vi "EventStructureLiftDev.vi"() -> ()   [LabVIEW 2016]
uses:
  <vilib>/myRIO/Instrument Drivers/Onboard IO/DIO/typedefs/DIO Reference.ctl
  <vilib>/myRIO/Common/Instrument Driver Framework/Utilities/typedefs/myRIO Generic Hardware Reference.ctl
  <vilib>/myRIO/Common/Instrument Driver Framework/Utilities/typedefs/Hardware Version Enum.ctl
  <vilib>/myRIO/Common/Instrument Driver Framework/Utilities/typedefs/myRIO v1.0 Reference.ctl
  <vilib>/myRIO/Common/Instrument Driver Framework/Utilities/typedefs/Generic FPGA Reference.ctl
  <vilib>/myRIO/Common/Instrument Driver Framework/myRIO v1.0/DIO/typedefs/DIO Channels List.ctl
  <vilib>/myRIO/Common/Instrument Driver Framework/myRIO v1.0/DIO/typedefs/DIO Channels Enum.ctl
  <vilib>/userdefined/High Color/nirio_resource_hc.ctl
  <vilib>/myRIO/Common/Instrument Driver Framework/Utilities/vis/Is FPGA Ref Available.vi
  <vilib>/myRIO/Common/Instrument Driver Framework/roboRIO v1.0/DIO/vis/roboRIO v1.0 Open DIO.vi
  <vilib>/myRIO/Instrument Drivers/Onboard IO/DIO/vis/Write.vi
  <vilib>/myRIO/Instrument Drivers/Onboard IO/DIO/vis/Read.vi
  <vilib>/myRIO/Common/Instrument Driver Framework/Utilities/vis/Validate Channels.vi
  <vilib>/myRIO/Common/Instrument Driver Framework/roboRIO v1.0/DIO/vis/roboRIO v1.0 Reserve DIO.vi
  <vilib>/myRIO/Common/Instrument Driver Framework/roboRIO v1.0/DIO/vis/roboRIO v1.0 Build MUX Configuration DIO.vi
  <vilib>/myRIO/Common/Instrument Driver Framework/roboRIO v1.0/Resource Manager/vis/roboRIO v1.0 Reserve Channel List.vi
  <vilib>/myRIO/Common/Instrument Driver Framework/roboRIO v1.0/Resource Manager/vis/roboRIO v1.0 Create Configuration List.vi
  <vilib>/myRIO/Common/Instrument Driver Framework/roboRIO v1.0/Resource Manager/vis/roboRIO v1.0 Reserve Channel.vi
  <vilib>/myRIO/Common/Instrument Driver Framework/roboRIO v1.0/Resource Manager/vis/roboRIO v1.0 Unreserve Channel.vi
  <vilib>/myRIO/Common/Instrument Driver Framework/roboRIO v1.0/Resource Manager/vis/roboRIO v1.0 Build Mutex Name.vi
  UnicornMain/GlobalVI.vi
  <vilib>/Utility/VariantDataType/GetNumericInfo.vi
  builds/UnicornMain/UnicornRIO1/ROS for LabVIEW/home/lvuser/natinst/bin/vi.lib/Utility/error.llb/Error Cluster From Error Code.vi
  <vilib>/myRIO/Common/Instrument Driver Framework/roboRIO v1.0/roboRIO v1.0 Open.vi
  <vilib>/myRIO/Common/Instrument Driver Framework/Utilities/vis/IO Manager.vi
  <vilib>/myRIO/Common/Instrument Driver Framework/Utilities/vis/Configuration Manager.vi
  <vilib>/myRIO/Common/Instrument Driver Framework/roboRIO v1.0/Resource Manager/vis/roboRIO v1.0 Configure IO.vi
  <vilib>/myRIO/Common/Instrument Driver Framework/myRIO v1.0/myRIO v1.0 Close.vi
  <vilib>/myRIO/Common/Instrument Driver Framework/roboRIO v1.0/DIO/vis/roboRIO v1.0 Write DIO.vi
  <vilib>/myRIO/Common/Instrument Driver Framework/roboRIO v1.0/DIO/vis/roboRIO v1.0 Read DIO.vi
  <vilib>/myRIO/Express VI/Onboard IO/DO/DO Express VI.xnode
  <vilib>/myRIO/Instrument Drivers/Onboard IO/DIO/vis/myRIO DIO Open.xnode
  <vilib>/myRIO/Express VI/Onboard Devices/LED/LED Express VI.xnode
  <vilib>/myRIO/Express VI/Onboard IO/DI/DI Express VI.xnode
  <vilib>/myRIO/Instrument Drivers/Onboard IO/DIO/DIO.lvlib
panel:
  out "UnloadBin":bool
  out "CancelBin":bool
  out "B/DIO7 (Pin 25) 2":bool
  out "B/DIO10 (Pin 31) 2":bool
  out "B/DIO10 (Pin 31) - Sensor 5\nBackwards 3":bool
  out "B/DIO7 (Pin 25) - Sensor 2 - Down 2":bool
  out "B/DIO9 (Pin 29) - Sensor4 - Forward 2":bool
  out "B/DIO8 (Pin 27) - Sensor3 - Up 2":bool
  out "LoadBin":bool
  out "B/DIO7 (Pin 25) - Sensor2 - Down 2":bool
  out "B/DIO10 (Pin 31) - Sensor 5\nBackwards 2":bool
  out "B/DIO8 (Pin 27) - Sensor 3 - Up 2":bool
  out "B/DIO9 (Pin 29) - Sensor 4 - Forward 2":bool
  out "StopBin":bool
  out "timeoutCounter":u32
  out "timeoutError":bool
  out "timerCount":u32
  out "liftState":i32
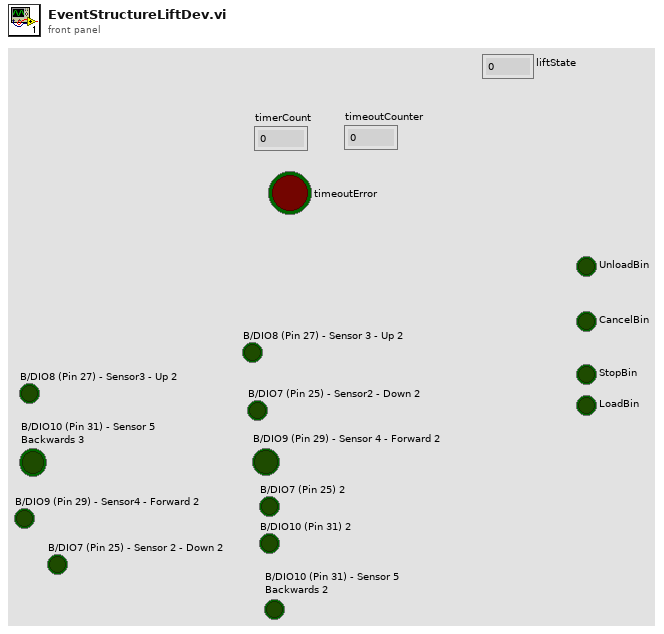
[diagram p1: front panel]
types:
  T1 = typedef "DIO.lvlib/DIO Reference.ctl" = cluster{"myRIO Reference":T2, "DIO Channels List":T6}
  T2 = typedef "myRIO Generic Hardware Reference.ctl" = cluster{"myRIO Model":T3, "myRIO Hardware Reference":T4}
  T3 = typedef "Hardware Version Enum.ctl" = enum16{"Unknown", "myRIO-1900", "myRIO-1950", "roboRIO", "NI ELVIS RIO CM"}
  T4 = typedef "myRIO v1.0 Reference.ctl" = cluster{"Generic FPGA Reference":T5, "Allow multiple opens":bool}
  T5 = typedef "Generic FPGA Reference.ctl" = refnum<k20>
  T6 = typedef "DIO Channels List.ctl" = T7[]
  T7 = typedef "DIO Channels Enum.ctl" = enum16{"Not Connected", "C/DIO0", "C/DIO1", "C/DIO2", "C/DIO3", "C/DIO4", "C/DIO5", "C/DIO6", "C/DIO7", "A/DIO0", "A/DIO1", "A/DIO2", "A/DIO3", "A/DIO4", "A/DIO5", "A/DIO6", "A/DIO7", "A/DIO8", "A/DIO9", "A/DIO10", "A/DIO11", "A/DIO12", "A/DIO13", "A/DIO14", "A/DIO15", "B/DIO0", "B/DIO1", "B/DIO2", "B/DIO3", "B/DIO4", "B/DIO5", "B/DIO6", "B/DIO7", "B/DIO8", "B/DIO9", "B/DIO10", "B/DIO11", "B/DIO12", "B/DIO13", "B/DIO14", "B/DIO15", "LED0", "LED1", "LED2", "LED3", "Button0", "DIO/DIO0", "DIO/DIO1", "DIO/DIO2", "DIO/DIO3", "DIO/DIO4", "DIO/DIO5", "DIO/DIO6", "DIO/DIO7", "DIO/DIO8", "DIO/DIO9", "SPI/CS0", "SPI/CS1", "SPI/CS2", "SPI/CS3", "LED RADIO (Green)", "LED RADIO (Red)", "LED COMM (Green)", "LED COMM (Red)", "LED MODE (Green)", "LED MODE (Red)"}
  T8 = typedef "nirio_resource_hc.ctl" = tag
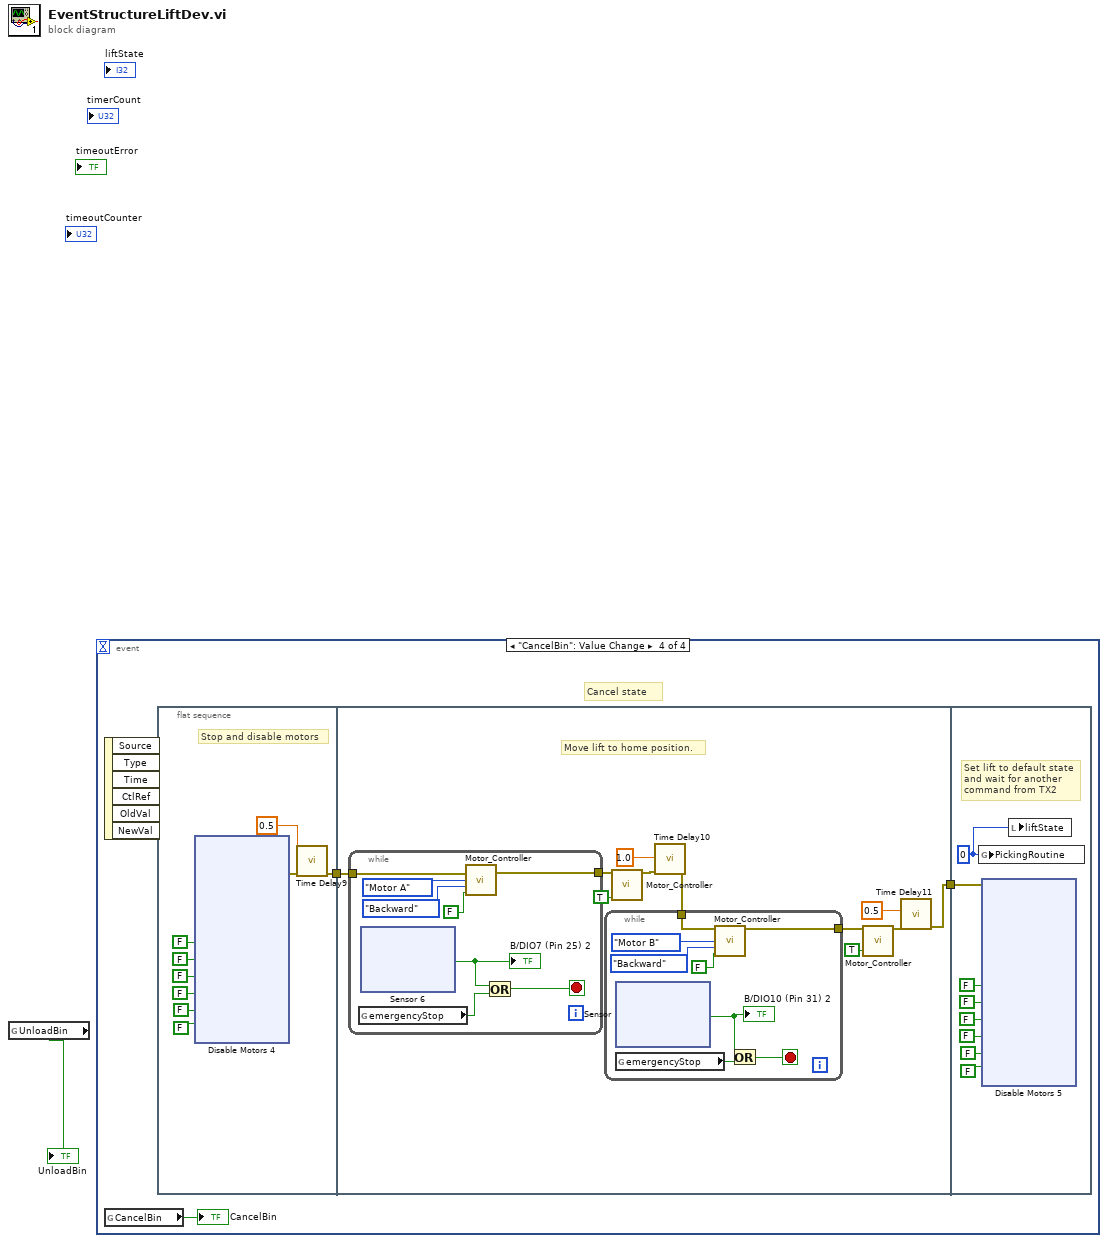
[diagram p0: block diagram]
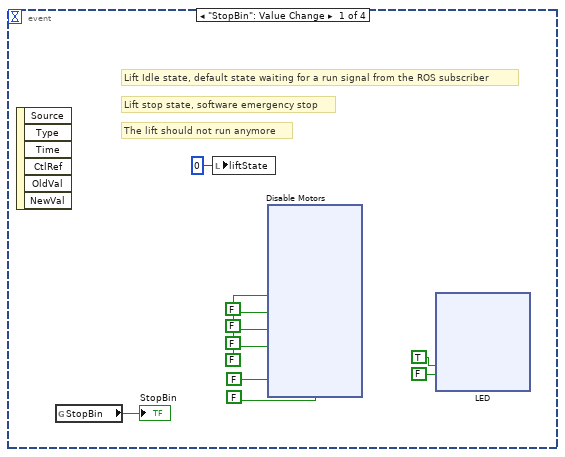
[diagram p2: hidden frame]
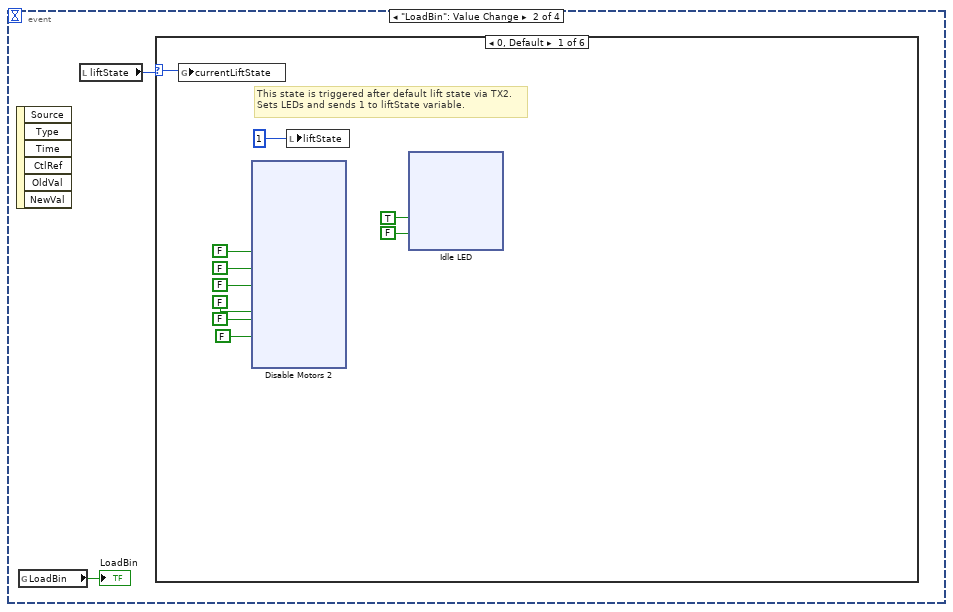
[diagram p3: hidden frame]
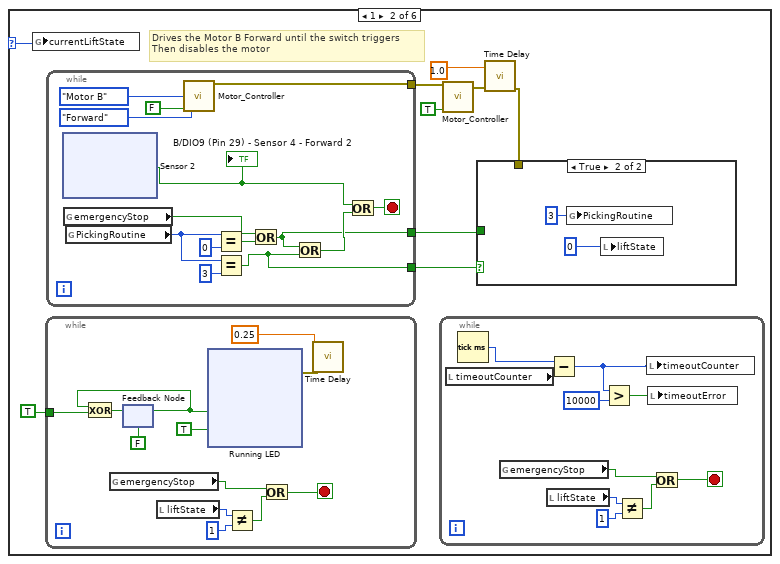
[diagram p4: hidden frame]
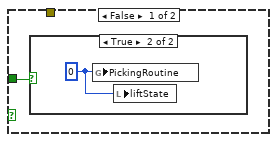
[diagram p5: hidden frame]
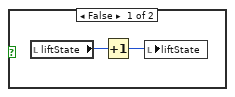
[diagram p6: hidden frame]
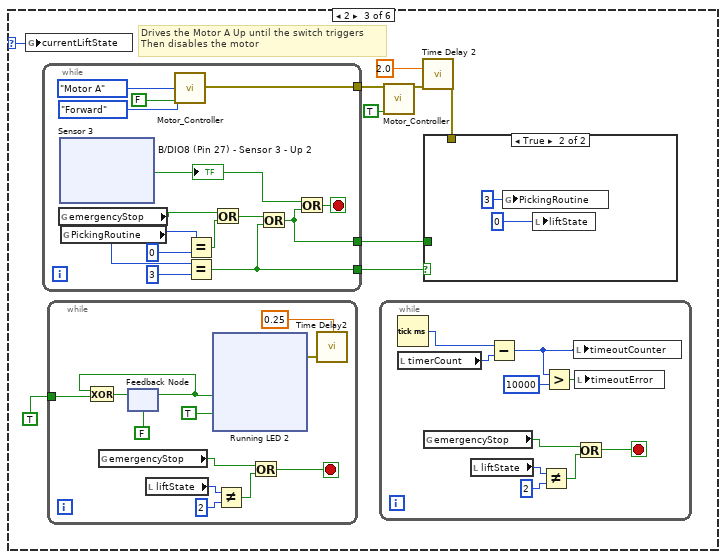
[diagram p7: hidden frame]
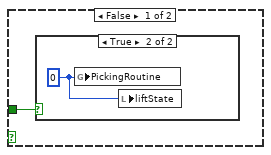
[diagram p8: hidden frame]
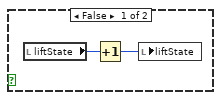
[diagram p9: hidden frame]
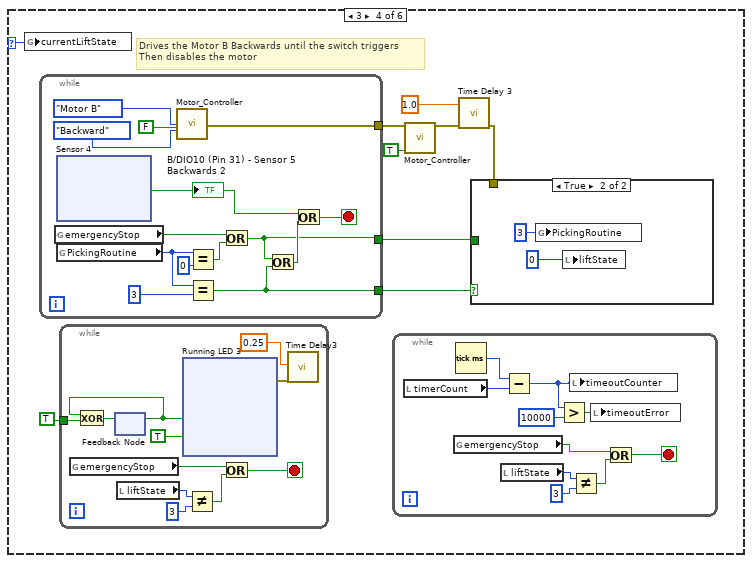
[diagram p10: hidden frame]
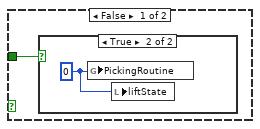
[diagram p11: hidden frame]
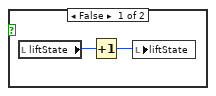
[diagram p12: hidden frame]
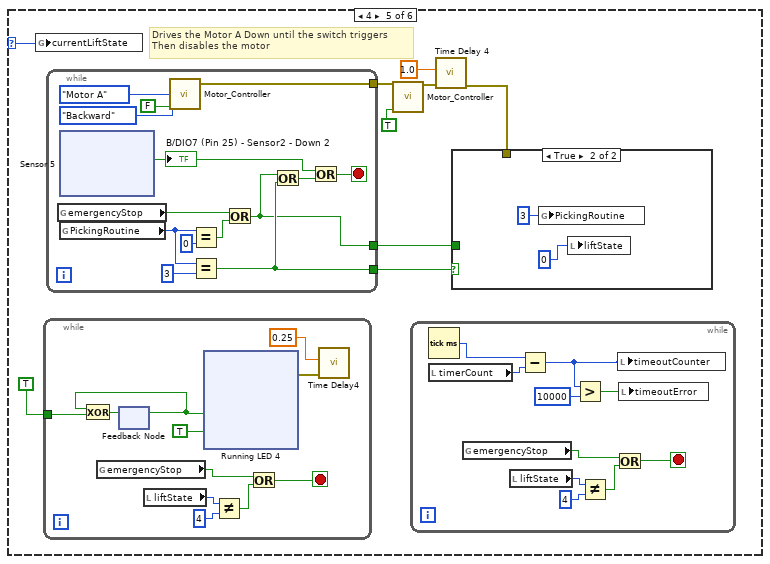
[diagram p13: hidden frame]
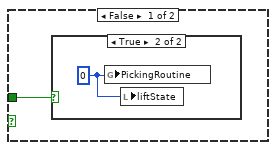
[diagram p14: hidden frame]
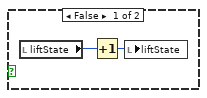
[diagram p15: hidden frame]
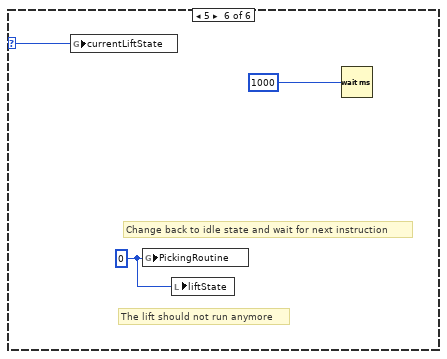
[diagram p16: hidden frame]
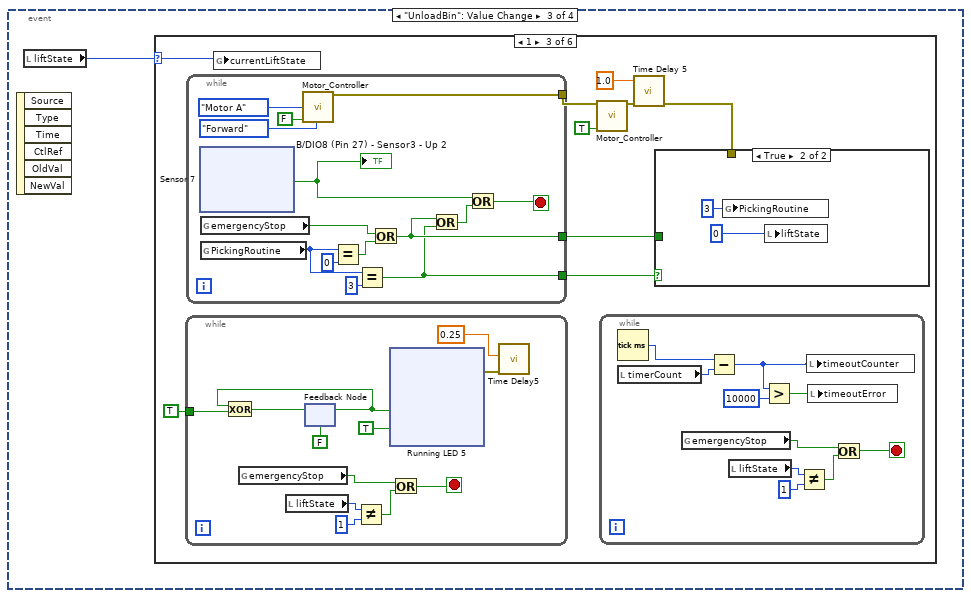
[diagram p17: hidden frame]
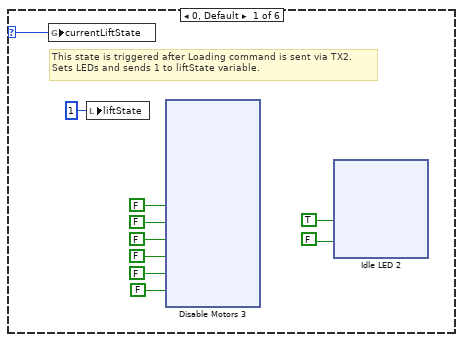
[diagram p18: hidden frame]
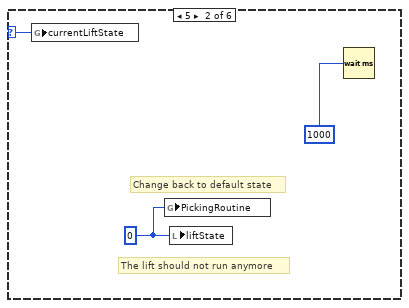
[diagram p19: hidden frame]
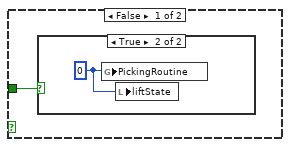
[diagram p20: hidden frame]
diagram:
  n1 = global read "GlobalVI.vi" "UnloadBin"() -> (→"UnloadBin":bool)
  n2 = event shown="[3] \"CancelBin\": Value Change" {
    selector: _ -> [_ _ _ _]
    dyn-events: _ -> [_ _ _ _]
    timeout: _ -> [_ _ _ _]
    event "StopBin": Value Change {
      # "Lift stop state, software emergency stop"
      # "Lift Idle state, default state waiting for a run signal from the ROS subscriber"
      # "The lift should not run anymore"
      n3 = event-data() -> ()  [unwired: 1 in, 6 out]
      n4 = global read "GlobalVI.vi" "StopBin"() -> (→"StopBin":bool)
      n5 = local write "liftState"(0 ("liftState")) -> ()
      n6 = xnode "Disable Motors"("IN1 (B/DIO1 (Pin 13))"=FALSE ("IN1 (B/DIO0 (Pin 11))"), "IN2 (B/DIO2 (Pin 15))"=FALSE ("IN2 (B/DIO1 (Pin 13))"), "IN3 (B/DIO4 (Pin 19))"=FALSE ("IN3 (B/DIO2 (Pin 15))"), "IN4 (B/DIO3 (Pin 17))"=FALSE, "ENABLE A (B/DIO0 (Pin 11))"=FALSE ("ENABLE A (B/DIO13 (Pin 26))"), "ENABLE B (B/DIO5 (Pin 21))"=FALSE ("ENABLE B (B/DIO8 (Pin 27))")) -> ()  [unwired: 1 in, 1 out]
      n7 = xnode "LED"("COMM (Green)"=TRUE, "COMM (Red)"=FALSE) -> ()  [unwired: 1 in, 1 out]
    }
    event "LoadBin": Value Change {
      n8 = event-data() -> ()  [unwired: 1 in, 6 out]
      n9 = global read "GlobalVI.vi" "LoadBin"() -> (→"LoadBin":bool)
      n10 = local read "liftState"() -> (w88:i32)
      n11 = case shown="0, Default" w88 {
        selector: w88 -> [w96 w179 w302 w423 w544 w664]
        frame 0, Default {
          # "This state is triggered after default lift state via TX2. \nSets LEDs and sends 1 to liftState variable."
          n12 = global write "GlobalVI.vi" "currentLiftState"(w96) -> ()
          n13 = xnode "Disable Motors 2"("IN1 (B/DIO1 (Pin 13))"=FALSE ("IN1 (B/DIO0 (Pin 11))"), "IN2 (B/DIO2 (Pin 15))"=FALSE ("IN2 (B/DIO1 (Pin 13))"), "IN3 (B/DIO4 (Pin 19))"=FALSE ("IN3 (B/DIO2 (Pin 15))"), "IN4 (B/DIO3 (Pin 17))"=FALSE, "ENABLE A (B/DIO0 (Pin 11))"=FALSE ("ENABLE A (B/DIO13 (Pin 26))"), "ENABLE B (B/DIO5 (Pin 21))"=FALSE ("ENABLE B (B/DIO8 (Pin 27))")) -> ()  [unwired: 1 in, 1 out]
          n14 = local write "liftState"(1 ("liftState")) -> ()
          n15 = xnode "Idle LED"("CommG"=TRUE, "CommR"=FALSE ("CommG")) -> ()  [unwired: 1 in, 1 out]
        }
        frame 1 {
          # "Drives the Motor B Forward until the switch triggers\nThen disables the motor"
          n16 = global write "GlobalVI.vi" "currentLiftState"(w179) -> ()
          n17 = while {
            tunnel: TRUE ("COMM (Red)") -> [w212]
            stop <- w202 stop-if-true
            n18 = global read "GlobalVI.vi" "emergencyStop"() -> (w203:bool)
            n19 = feedback #1(FALSE) -> (w210:bool)
            n20 = Exclusive Or(1:w212, 2:w210) -> (0:w211:bool)
            n21 = feedback-in #1(w211) -> ()
            n22 = local read "liftState"() -> (w205:i32)
            n23 = xnode "Running LED"("CommG"=w210, "CommR"=TRUE) -> ("error out"=w207:errorcluster)  [unwired: 1 in]
            n24 = Not Equal?(x=w205, y=1 ("liftState")) -> (x != y?=w204:bool)
            n25 = Or(x=w203, y=w204) -> (x .or. y?=w202:bool)
            n26 = call "Time Delay"("error in (no error)"=w207, "Delay Time (s)"=0.25) -> ()  [unwired: 9 in, 1 out]
          }
          n27 = while {
            tunnel: [w261] -> w180
            tunnel: [w250] -> w177
            tunnel: [w249] -> w178
            stop <- w262 stop-if-true
            n28 = xnode "Sensor 2"() -> ("B/DIO9 (Pin 29)"=w257:bool)  [unwired: 1 in, 1 out]
            "B/DIO9 (Pin 29) - Sensor 4 - Forward 2" <- w257
            n29 = global read "GlobalVI.vi" "emergencyStop"() -> (w255:bool)
            n30 = global read "GlobalVI.vi" "PickingRoutine"() -> (w252:i32)
            n31 = call "Motor_Controller.vi"("motorSelect"=enum16{"Motor A", "Motor B"}."Motor B", "direction"=enum16{"Forward", "Backward"}."Forward", "stopMotors"=FALSE) -> ("error out"=w261:errorcluster)  [unwired: 12 in]
            n32 = Equal?(x=w252, y=0) -> (x = y?=w254:bool)
            n33 = Equal?(x=w252, y=3) -> (x = y?=w249:bool)
            n34 = Or(x=w255, y=w254) -> (x .or. y?=w250:bool)
            n35 = Or(x=w250, y=w249) -> (x .or. y?=w251:bool)
            n36 = Or(x=w257, y=w251) -> (x .or. y?=w262:bool)
          }
          n37 = while {
            stop <- w194 stop-if-true
            n38 = local read "timeoutCounter"() -> (w199:u32)
            n39 = Tick Count (ms)() -> (millisecond timer value=w200:u32)
            n40 = global read "GlobalVI.vi" "emergencyStop"() -> (w198:bool)
            n41 = local read "liftState"() -> (w196:i32)
            n42 = Subtract(x=w200, y=w199) -> (x-y=w191:u32)
            n43 = Greater?(x=w191, y=u32 10000) -> (0:w192:bool)
            n44 = Not Equal?(x=w196, y=1 ("liftState")) -> (x != y?=w197:bool)
            n45 = local write "timeoutCounter"(w191) -> ()
            n46 = local write "timeoutError"(w192) -> ()
            n47 = Or(x=w198, y=w197) -> (x .or. y?=w194:bool)
          }
          n48 = call "Motor_Controller.vi"("error in (no error)"=w180, "stopMotors"=TRUE) -> ("error out"=w181:errorcluster)  [unwired: 13 in]
          n49 = call "Time Delay"("error in (no error)"=w181, "Delay Time (s)"=1.0) -> ("error out"=w176:errorcluster)  [unwired: 9 in]
          n50 = case shown="True" w178 {
            tunnel: w177 -> [w185 _]
            tunnel: w176 -> [_ _]
            frame False {
              n51 = case shown="True" w185 {
                frame False {
                  n52 = local read "liftState"() -> (w187:i32)
                  n53 = Increment(x=w187) -> (x+1=w186:i32)
                  n54 = local write "liftState"(w186) -> ()
                }
                frame True {
                  w188 = 0 ("liftState")
                  n55 = global write "GlobalVI.vi" "PickingRoutine"(w188) -> ()
                  n56 = local write "liftState"(w188) -> ()
                }
              }
            }
            frame True {
              n57 = global write "GlobalVI.vi" "PickingRoutine"(3 ("PickingRoutine")) -> ()
              n58 = local write "liftState"(0 ("liftState")) -> ()
            }
          }
        }
        frame 2 {
          # "Drives the Motor A Up until the switch triggers\nThen disables the motor"
          n59 = global write "GlobalVI.vi" "currentLiftState"(w302) -> ()
          n60 = while {
            tunnel: [w382] -> w301
            tunnel: [w372] -> w300
            tunnel: [w371] -> w299
            stop <- w379 stop-if-true
            n61 = global read "GlobalVI.vi" "emergencyStop"() -> (w378:bool)
            n62 = xnode "Sensor 3"() -> ("Upwards (B/DIO8 (Pin 27))"=w380:bool)  [unwired: 1 in, 1 out]
            "B/DIO8 (Pin 27) - Sensor 3 - Up 2" <- w380
            n63 = global read "GlobalVI.vi" "PickingRoutine"() -> (w374:i32)
            n64 = call "Motor_Controller.vi"("motorSelect"=enum16{"Motor A", "Motor B"}."Motor A", "direction"=enum16{"Forward", "Backward"}."Forward", "stopMotors"=FALSE) -> ("error out"=w382:errorcluster)  [unwired: 12 in]
            n65 = Equal?(x=w374, y=0) -> (x = y?=w377:bool)
            n66 = Equal?(x=w374, y=3) -> (x = y?=w372:bool)
            n67 = Or(x=w378, y=w377) -> (x .or. y?=w373:bool)
            n68 = Or(x=w373, y=w372) -> (x .or. y?=w371:bool)
            n69 = Or(x=w380, y=w371) -> (x .or. y?=w379:bool)
          }
          n70 = while {
            tunnel: TRUE ("COMM (Red)") -> [w334]
            stop <- w324 stop-if-true
            n71 = global read "GlobalVI.vi" "emergencyStop"() -> (w325:bool)
            n72 = feedback #2(FALSE) -> (w332:bool)
            n73 = Exclusive Or(1:w334, 2:w332) -> (0:w333:bool)
            n74 = feedback-in #2(w333) -> ()
            n75 = local read "liftState"() -> (w327:i32)
            n76 = xnode "Running LED 2"("CommG"=w332, "CommR"=TRUE) -> ("error out"=w329:errorcluster)  [unwired: 1 in]
            n77 = Not Equal?(x=w327, y=2 ("liftState")) -> (x != y?=w326:bool)
            n78 = Or(x=w325, y=w326) -> (x .or. y?=w324:bool)
            n79 = call "Time Delay2"("error in (no error)"=w329, "Delay Time (s)"=0.25) -> ()  [unwired: 9 in, 1 out]
          }
          n80 = while {
            stop <- w316 stop-if-true
            n81 = Tick Count (ms)() -> (millisecond timer value=w322:u32)
            n82 = local read "timerCount"() -> (w321:u32)
            n83 = global read "GlobalVI.vi" "emergencyStop"() -> (w320:bool)
            n84 = local read "liftState"() -> (w318:i32)
            n85 = Subtract(x=w322, y=w321) -> (x-y=w313:u32)
            n86 = Not Equal?(x=w318, y=2 ("liftState")) -> (x != y?=w319:bool)
            n87 = Greater?(x=w313, y=u32 10000) -> (0:w314:bool)
            n88 = local write "timeoutCounter"(w313) -> ()
            n89 = local write "timeoutError"(w314) -> ()
            n90 = Or(x=w320, y=w319) -> (x .or. y?=w316:bool)
          }
          n91 = call "Motor_Controller.vi"("error in (no error)"=w301, "stopMotors"=TRUE) -> ("error out"=w303:errorcluster)  [unwired: 13 in]
          n92 = call "Time Delay 2"("error in (no error)"=w303, "Delay Time (s)"=2.0) -> ("error out"=w298:errorcluster)  [unwired: 9 in]
          n93 = case shown="True" w300 {
            tunnel: w299 -> [w307 _]
            tunnel: w298 -> [_ _]
            frame False {
              n94 = case shown="True" w307 {
                frame False {
                  n95 = local read "liftState"() -> (w309:i32)
                  n96 = Increment(x=w309) -> (x+1=w308:i32)
                  n97 = local write "liftState"(w308) -> ()
                }
                frame True {
                  w310 = 0 ("liftState")
                  n98 = global write "GlobalVI.vi" "PickingRoutine"(w310) -> ()
                  n99 = local write "liftState"(w310) -> ()
                }
              }
            }
            frame True {
              n100 = global write "GlobalVI.vi" "PickingRoutine"(3 ("PickingRoutine")) -> ()
              n101 = local write "liftState"(0 ("liftState")) -> ()
            }
          }
        }
        frame 3 {
          # "Drives the Motor B Backwards until the switch triggers\nThen disables the motor"
          n102 = global write "GlobalVI.vi" "currentLiftState"(w423) -> ()
          n103 = while {
            tunnel: [w493] -> w422
            tunnel: [w502] -> w425
            tunnel: [w492] -> w421
            stop <- w505 stop-if-true
            n104 = global read "GlobalVI.vi" "emergencyStop"() -> (w498:bool)
            n105 = xnode "Sensor 4"() -> ("B/DIO10 (Pin 31)"=w500:bool)  [unwired: 1 in, 1 out]
            "B/DIO10 (Pin 31) - Sensor 5\nBackwards 2" <- w500
            n106 = global read "GlobalVI.vi" "PickingRoutine"() -> (w496:i32)
            n107 = call "Motor_Controller.vi"("motorSelect"=enum16{"Motor A", "Motor B"}."Motor B", "direction"=enum16{"Forward", "Backward"}."Backward", "stopMotors"=FALSE) -> ("error out"=w502:errorcluster)  [unwired: 12 in]
            n108 = Equal?(x=w496, y=0) -> (x = y?=w497:bool)
            n109 = Equal?(x=w496, y=3) -> (x = y?=w493:bool)
            n110 = Or(x=w498, y=w497) -> (x .or. y?=w492:bool)
            n111 = Or(x=w492, y=w493) -> (x .or. y?=w494:bool)
            n112 = Or(x=w500, y=w494) -> (x .or. y?=w505:bool)
          }
          n113 = while {
            tunnel: TRUE ("COMM (Red)") -> [w455]
            stop <- w445 stop-if-true
            n114 = global read "GlobalVI.vi" "emergencyStop"() -> (w446:bool)
            n115 = feedback #3() -> (w453:bool)  [unwired: 1 in]
            n116 = Exclusive Or(1:w455, 2:w453) -> (0:w454:bool)
            n117 = feedback-in #3(w454) -> ()
            n118 = local read "liftState"() -> (w448:i32)
            n119 = xnode "Running LED 3"("CommG"=w453, "CommR"=TRUE) -> ("error out"=w450:errorcluster)  [unwired: 1 in]
            n120 = Not Equal?(x=w448, y=3 ("liftState")) -> (x != y?=w447:bool)
            n121 = Or(x=w446, y=w447) -> (x .or. y?=w445:bool)
            n122 = call "Time Delay3"("error in (no error)"=w450, "Delay Time (s)"=0.25) -> ()  [unwired: 9 in, 1 out]
          }
          n123 = while {
            stop <- w438 stop-if-true
            n124 = local read "timerCount"() -> (w443:u32)
            n125 = global read "GlobalVI.vi" "emergencyStop"() -> (w442:bool)
            n126 = Tick Count (ms)() -> (millisecond timer value=w444:u32)
            n127 = local read "liftState"() -> (w440:i32)
            n128 = Subtract(x=w444, y=w443) -> (x-y=w435:u32)
            n129 = Greater?(x=w435, y=u32 10000) -> (0:w436:bool)
            n130 = local write "timeoutCounter"(w435) -> ()
            n131 = Not Equal?(x=w440, y=3 ("liftState")) -> (x != y?=w441:bool)
            n132 = local write "timeoutError"(w436) -> ()
            n133 = Or(x=w442, y=w441) -> (x .or. y?=w438:bool)
          }
          n134 = call "Motor_Controller.vi"("error in (no error)"=w425, "stopMotors"=TRUE) -> ("error out"=w424:errorcluster)  [unwired: 13 in]
          n135 = call "Time Delay 3"("error in (no error)"=w424, "Delay Time (s)"=1.0) -> ("error out"=w420:errorcluster)  [unwired: 9 in]
          n136 = case shown="True" w422 {
            tunnel: w421 -> [w429 _]
            tunnel: w420 -> [_ _]
            frame False {
              n137 = case shown="True" w429 {
                frame False {
                  n138 = local read "liftState"() -> (w431:i32)
                  n139 = Increment(x=w431) -> (x+1=w430:i32)
                  n140 = local write "liftState"(w430) -> ()
                }
                frame True {
                  w432 = 0 ("liftState")
                  n141 = global write "GlobalVI.vi" "PickingRoutine"(w432) -> ()
                  n142 = local write "liftState"(w432) -> ()
                }
              }
            }
            frame True {
              n143 = global write "GlobalVI.vi" "PickingRoutine"(3 ("PickingRoutine")) -> ()
              n144 = local write "liftState"(0 ("liftState")) -> ()
            }
          }
        }
        frame 4 {
          # "Drives the Motor A Down until the switch triggers\nThen disables the motor"
          n145 = global write "GlobalVI.vi" "currentLiftState"(w544) -> ()
          n146 = while {
            tunnel: TRUE ("COMM (Red)") -> [w576]
            stop <- w566 stop-if-true
            n147 = global read "GlobalVI.vi" "emergencyStop"() -> (w567:bool)
            n148 = feedback #4() -> (w574:bool)  [unwired: 1 in]
            n149 = Exclusive Or(1:w576, 2:w574) -> (0:w575:bool)
            n150 = feedback-in #4(w575) -> ()
            n151 = local read "liftState"() -> (w569:i32)
            n152 = xnode "Running LED 4"("CommG"=w574, "CommR"=TRUE) -> ("error out"=w571:errorcluster)  [unwired: 1 in]
            n153 = Not Equal?(x=w569, y=4 ("liftState")) -> (x != y?=w568:bool)
            n154 = Or(x=w567, y=w568) -> (x .or. y?=w566:bool)
            n155 = call "Time Delay4"("error in (no error)"=w571, "Delay Time (s)"=0.25) -> ()  [unwired: 9 in, 1 out]
          }
          n156 = while {
            tunnel: [w623] -> w546
            tunnel: [w616] -> w543
            tunnel: [w614] -> w542
            stop <- w626 stop-if-true
            n157 = global read "GlobalVI.vi" "emergencyStop"() -> (w619:bool)
            n158 = xnode "Sensor 5"() -> ("B/DIO7 (Pin 25)"=w621:bool)  [unwired: 1 in, 1 out]
            "B/DIO7 (Pin 25) - Sensor2 - Down 2" <- w621
            n159 = global read "GlobalVI.vi" "PickingRoutine"() -> (w617:i32)
            n160 = call "Motor_Controller.vi"("motorSelect"=enum16{"Motor A", "Motor B"}."Motor A", "direction"=enum16{"Forward", "Backward"}."Backward", "stopMotors"=FALSE) -> ("error out"=w623:errorcluster)  [unwired: 12 in]
            n161 = Equal?(x=w617, y=0) -> (x = y?=w618:bool)
            n162 = Equal?(x=w617, y=3) -> (x = y?=w616:bool)
            n163 = Or(x=w619, y=w618) -> (x .or. y?=w614:bool)
            n164 = Or(x=w614, y=w616) -> (x .or. y?=w615:bool)
            n165 = Or(x=w621, y=w615) -> (x .or. y?=w626:bool)
          }
          n166 = call "Motor_Controller.vi"("error in (no error)"=w546, "stopMotors"=TRUE) -> ("error out"=w545:errorcluster)  [unwired: 13 in]
          n167 = while {
            stop <- w559 stop-if-true
            n168 = Tick Count (ms)() -> (millisecond timer value=w565:u32)
            n169 = local read "timerCount"() -> (w564:u32)
            n170 = global read "GlobalVI.vi" "emergencyStop"() -> (w563:bool)
            n171 = local read "liftState"() -> (w561:i32)
            n172 = Subtract(x=w565, y=w564) -> (x-y=w556:u32)
            n173 = Greater?(x=w556, y=u32 10000) -> (0:w557:bool)
            n174 = Not Equal?(x=w561, y=4 ("liftState")) -> (x != y?=w562:bool)
            n175 = Or(x=w563, y=w562) -> (x .or. y?=w559:bool)
            n176 = local write "timeoutCounter"(w556) -> ()
            n177 = local write "timeoutError"(w557) -> ()
          }
          n178 = call "Time Delay 4"("error in (no error)"=w545, "Delay Time (s)"=1.0) -> ("error out"=w541:errorcluster)  [unwired: 9 in]
          n179 = case shown="True" w543 {
            tunnel: w542 -> [w550 _]
            tunnel: w541 -> [_ _]
            frame False {
              n180 = case shown="True" w550 {
                frame False {
                  n181 = local read "liftState"() -> (w552:i32)
                  n182 = Increment(x=w552) -> (x+1=w551:i32)
                  n183 = local write "liftState"(w551) -> ()
                }
                frame True {
                  w553 = 0 ("liftState")
                  n184 = global write "GlobalVI.vi" "PickingRoutine"(w553) -> ()
                  n185 = local write "liftState"(w553) -> ()
                }
              }
            }
            frame True {
              n186 = global write "GlobalVI.vi" "PickingRoutine"(3 ("PickingRoutine")) -> ()
              n187 = local write "liftState"(0 ("liftState")) -> ()
            }
          }
        }
        frame 5 {
          w662 = 0 ("liftState")
          # "The lift should not run anymore"
          # "Change back to idle state and wait for next instruction"
          n188 = global write "GlobalVI.vi" "currentLiftState"(w664) -> ()
          n189 = global write "GlobalVI.vi" "PickingRoutine"(w662) -> ()
          n190 = local write "liftState"(w662) -> ()
          n191 = Wait (ms)(milliseconds to wait=u32 1000) -> ()  [unwired: 1 out]
        }
      }
    }
    event "UnloadBin": Value Change {
      n192 = event-data() -> ()  [unwired: 1 in, 6 out]
      n193 = local read "liftState"() -> (w665:i32)
      n194 = case shown="1" w665 {
        selector: w665 -> [w672 w754 w763 w880 w1002 w1124]
        frame 0, Default {
          # "This state is triggered after Loading command is sent via TX2. \nSets LEDs and sends 1 to liftState variable."
          n195 = global write "GlobalVI.vi" "currentLiftState"(w672) -> ()
          n196 = local write "liftState"(1 ("liftState")) -> ()
          n197 = xnode "Disable Motors 3"("IN1 (B/DIO1 (Pin 13))"=FALSE ("IN1 (B/DIO0 (Pin 11))"), "IN2 (B/DIO2 (Pin 15))"=FALSE ("IN2 (B/DIO1 (Pin 13))"), "IN3 (B/DIO4 (Pin 19))"=FALSE ("IN3 (B/DIO2 (Pin 15))"), "IN4 (B/DIO3 (Pin 17))"=FALSE, "ENABLE A (B/DIO0 (Pin 11))"=FALSE ("ENABLE A (B/DIO13 (Pin 26))"), "ENABLE B (B/DIO5 (Pin 21))"=FALSE ("ENABLE B (B/DIO8 (Pin 27))")) -> ()  [unwired: 1 in, 1 out]
          n198 = xnode "Idle LED 2"("CommG"=TRUE, "CommR"=FALSE ("CommG")) -> ()  [unwired: 1 in, 1 out]
        }
        frame 5 {
          w752 = 0 ("liftState")
          # "The lift should not run anymore"
          # "Change back to default state"
          n199 = global write "GlobalVI.vi" "currentLiftState"(w754) -> ()
          n200 = global write "GlobalVI.vi" "PickingRoutine"(w752) -> ()
          n201 = local write "liftState"(w752) -> ()
          n202 = Wait (ms)(milliseconds to wait=u32 1000) -> ()  [unwired: 1 out]
        }
        frame 1 {
          n203 = while {
            tunnel: TRUE ("COMM (Red)") -> [w791]
            stop <- w781 stop-if-true
            n204 = global read "GlobalVI.vi" "emergencyStop"() -> (w782:bool)
            n205 = local read "liftState"() -> (w784:i32)
            n206 = feedback #5(FALSE) -> (w789:bool)
            n207 = Exclusive Or(1:w791, 2:w789) -> (0:w790:bool)
            n208 = feedback-in #5(w790) -> ()
            n209 = Not Equal?(x=w784, y=1 ("liftState")) -> (x != y?=w783:bool)
            n210 = xnode "Running LED 5"("CommG"=w789, "CommR"=TRUE) -> ("error out"=w786:errorcluster)  [unwired: 1 in]
            n211 = Or(x=w782, y=w783) -> (x .or. y?=w781:bool)
            n212 = call "Time Delay5"("error in (no error)"=w786, "Delay Time (s)"=0.25) -> ()  [unwired: 9 in, 1 out]
          }
          n213 = while {
            tunnel: [w840] -> w758
            tunnel: [w831] -> w755
            tunnel: [w828] -> w756
            stop <- w841 stop-if-true
            n214 = xnode "Sensor 7"() -> ("B/DIO8 (Pin 27)"=w836:bool)  [unwired: 1 in, 1 out]
            "B/DIO8 (Pin 27) - Sensor3 - Up 2" <- w836
            n215 = global read "GlobalVI.vi" "emergencyStop"() -> (w833:bool)
            n216 = global read "GlobalVI.vi" "PickingRoutine"() -> (w830:i32)
            n217 = call "Motor_Controller.vi"("motorSelect"=enum16{"Motor A", "Motor B"}."Motor A", "direction"=enum16{"Forward", "Backward"}."Forward", "stopMotors"=FALSE) -> ("error out"=w840:errorcluster)  [unwired: 12 in]
            n218 = Equal?(x=w830, y=0) -> (x = y?=w834:bool)
            n219 = Equal?(x=w830, y=3) -> (x = y?=w828:bool)
            n220 = Or(x=w833, y=w834) -> (x .or. y?=w831:bool)
            n221 = Or(x=w831, y=w828) -> (x .or. y?=w829:bool)
            n222 = Or(x=w836, y=w829) -> (x .or. y?=w841:bool)
          }
          n223 = global write "GlobalVI.vi" "currentLiftState"(w763) -> ()
          n224 = call "Motor_Controller.vi"("error in (no error)"=w758, "stopMotors"=TRUE) -> ("error out"=w759:errorcluster)  [unwired: 13 in]
          n225 = while {
            stop <- w773 stop-if-true
            n226 = Tick Count (ms)() -> (millisecond timer value=w779:u32)
            n227 = local read "timerCount"() -> (w778:u32)
            n228 = global read "GlobalVI.vi" "emergencyStop"() -> (w777:bool)
            n229 = Subtract(x=w779, y=w778) -> (x-y=w770:u32)
            n230 = local read "liftState"() -> (w775:i32)
            n231 = Greater?(x=w770, y=u32 10000) -> (0:w771:bool)
            n232 = Not Equal?(x=w775, y=1 ("liftState")) -> (x != y?=w776:bool)
            n233 = local write "timeoutCounter"(w770) -> ()
            n234 = local write "timeoutError"(w771) -> ()
            n235 = Or(x=w777, y=w776) -> (x .or. y?=w773:bool)
          }
          n236 = call "Time Delay 5"("error in (no error)"=w759, "Delay Time (s)"=1.0) -> ("error out"=w757:errorcluster)  [unwired: 9 in]
          n237 = case shown="True" w756 {
            tunnel: w757 -> [_ _]
            tunnel: w755 -> [w764 _]
            frame False {
              n238 = case shown="True" w764 {
                frame False {
                  n239 = local read "liftState"() -> (w766:i32)
                  n240 = Increment(x=w766) -> (x+1=w765:i32)
                  n241 = local write "liftState"(w765) -> ()
                }
                frame True {
                  w767 = 0 ("liftState")
                  n242 = global write "GlobalVI.vi" "PickingRoutine"(w767) -> ()
                  n243 = local write "liftState"(w767) -> ()
                }
              }
            }
            frame True {
              n244 = global write "GlobalVI.vi" "PickingRoutine"(3 ("PickingRoutine")) -> ()
              n245 = local write "liftState"(0 ("liftState")) -> ()
            }
          }
        }
        frame 2 {
          n246 = while {
            tunnel: TRUE ("COMM (Red)") -> [w913]
            stop <- w903 stop-if-true
            n247 = feedback #6(FALSE) -> (w911:bool)
            n248 = Exclusive Or(1:w913, 2:w911) -> (0:w912:bool)
            n249 = feedback-in #6(w912) -> ()
            n250 = global read "GlobalVI.vi" "emergencyStop"() -> (w904:bool)
            n251 = local read "liftState"() -> (w906:i32)
            n252 = xnode "Running LED 6"("CommG"=w911, "CommR"=TRUE) -> ("error out"=w908:errorcluster)  [unwired: 1 in]
            n253 = Not Equal?(x=w906, y=2 ("liftState")) -> (x != y?=w905:bool)
            n254 = Or(x=w904, y=w905) -> (x .or. y?=w903:bool)
            n255 = call "Time Delay6"("error in (no error)"=w908, "Delay Time (s)"=0.25) -> ()  [unwired: 9 in, 1 out]
          }
          n256 = while {
            tunnel: [w962] -> w881
            tunnel: [w952] -> w878
            tunnel: [w950] -> w879
            stop <- w963 stop-if-true
            n257 = xnode "Sensor 8"() -> ("B/DIO9 (Pin 29)"=w958:bool)  [unwired: 1 in, 1 out]
            "B/DIO9 (Pin 29) - Sensor4 - Forward 2" <- w958
            n258 = global read "GlobalVI.vi" "emergencyStop"() -> (w955:bool)
            n259 = global read "GlobalVI.vi" "PickingRoutine"() -> (w953:i32)
            n260 = call "Motor_Controller.vi"("motorSelect"=enum16{"Motor A", "Motor B"}."Motor B", "direction"=enum16{"Forward", "Backward"}."Forward", "stopMotors"=FALSE) -> ("error out"=w962:errorcluster)  [unwired: 12 in]
            n261 = Equal?(x=w953, y=0) -> (x = y?=w956:bool)
            n262 = Equal?(x=w953, y=3) -> (x = y?=w950:bool)
            n263 = Or(x=w955, y=w956) -> (x .or. y?=w952:bool)
            n264 = Or(x=w952, y=w950) -> (x .or. y?=w951:bool)
            n265 = Or(x=w958, y=w951) -> (x .or. y?=w963:bool)
          }
          n266 = global write "GlobalVI.vi" "currentLiftState"(w880) -> ()
          n267 = call "Motor_Controller.vi"("error in (no error)"=w881, "stopMotors"=TRUE) -> ("error out"=w882:errorcluster)  [unwired: 13 in]
          n268 = while {
            stop <- w895 stop-if-true
            n269 = Tick Count (ms)() -> (millisecond timer value=w901:u32)
            n270 = local read "timerCount"() -> (w900:u32)
            n271 = global read "GlobalVI.vi" "emergencyStop"() -> (w899:bool)
            n272 = Subtract(x=w901, y=w900) -> (x-y=w892:u32)
            n273 = local read "liftState"() -> (w897:i32)
            n274 = Greater?(x=w892, y=u32 10000) -> (0:w893:bool)
            n275 = Not Equal?(x=w897, y=2 ("liftState")) -> (x != y?=w898:bool)
            n276 = local write "timeoutCounter"(w892) -> ()
            n277 = local write "timeoutError"(w893) -> ()
            n278 = Or(x=w899, y=w898) -> (x .or. y?=w895:bool)
          }
          n279 = call "Time Delay 6"("error in (no error)"=w882, "Delay Time (s)"=1.0) -> ("error out"=w877:errorcluster)  [unwired: 9 in]
          n280 = case shown="True" w879 {
            tunnel: w878 -> [w886 _]
            tunnel: w877 -> [_ _]
            frame False {
              n281 = case shown="True" w886 {
                frame False {
                  n282 = local read "liftState"() -> (w888:i32)
                  n283 = Increment(x=w888) -> (x+1=w887:i32)
                  n284 = local write "liftState"(w887) -> ()
                }
                frame True {
                  w889 = 0 ("PickingRoutine")
                  n285 = global write "GlobalVI.vi" "PickingRoutine"(w889) -> ()
                  n286 = local write "liftState"(w889) -> ()
                }
              }
            }
            frame True {
              n287 = global write "GlobalVI.vi" "PickingRoutine"(3 ("PickingRoutine")) -> ()
              n288 = local write "liftState"(0 ("liftState")) -> ()
            }
          }
        }
        frame 3 {
          n289 = while {
            tunnel: TRUE ("COMM (Red)") -> [w1035]
            stop <- w1025 stop-if-true
            n290 = feedback #7(FALSE) -> (w1033:bool)
            n291 = Exclusive Or(1:w1035, 2:w1033) -> (0:w1034:bool)
            n292 = feedback-in #7(w1034) -> ()
            n293 = global read "GlobalVI.vi" "emergencyStop"() -> (w1026:bool)
            n294 = xnode "Running LED 7"("CommG"=w1033, "CommR"=TRUE) -> ("error out"=w1030:errorcluster)  [unwired: 1 in]
            n295 = local read "liftState"() -> (w1028:i32)
            n296 = Not Equal?(x=w1028, y=3 ("liftState")) -> (x != y?=w1027:bool)
            n297 = Or(x=w1026, y=w1027) -> (x .or. y?=w1025:bool)
            n298 = call "Time Delay7"("error in (no error)"=w1030, "Delay Time (s)"=0.25) -> ()  [unwired: 9 in, 1 out]
          }
          n299 = while {
            tunnel: [w1085] -> w1003
            tunnel: [w1073] -> w1000
            tunnel: [w1072] -> w999
            stop <- w1080 stop-if-true
            n300 = xnode "Sensor 9"() -> ("Downwards (B/DIO7 (Pin 25))"=w1081:bool)  [unwired: 1 in, 1 out]
            "B/DIO7 (Pin 25) - Sensor 2 - Down 2" <- w1081
            n301 = global read "GlobalVI.vi" "emergencyStop"() -> (w1078:bool)
            n302 = global read "GlobalVI.vi" "PickingRoutine"() -> (w1075:i32)
            n303 = call "Motor_Controller.vi"("motorSelect"=enum16{"Motor A", "Motor B"}."Motor A", "direction"=enum16{"Forward", "Backward"}."Backward", "stopMotors"=FALSE) -> ("error out"=w1085:errorcluster)  [unwired: 12 in]
            n304 = Equal?(x=w1075, y=0) -> (x = y?=w1077:bool)
            n305 = Equal?(x=w1075, y=3) -> (x = y?=w1072:bool)
            n306 = Or(x=w1078, y=w1077) -> (x .or. y?=w1073:bool)
            n307 = Or(x=w1073, y=w1072) -> (x .or. y?=w1074:bool)
            n308 = Or(x=w1081, y=w1074) -> (x .or. y?=w1080:bool)
          }
          n309 = global write "GlobalVI.vi" "currentLiftState"(w1002) -> ()
          n310 = call "Motor_Controller.vi"("error in (no error)"=w1003, "stopMotors"=TRUE) -> ("error out"=w1004:errorcluster)  [unwired: 13 in]
          n311 = while {
            stop <- w1017 stop-if-true
            n312 = Tick Count (ms)() -> (millisecond timer value=w1023:u32)
            n313 = local read "timerCount"() -> (w1022:u32)
            n314 = Subtract(x=w1023, y=w1022) -> (x-y=w1014:u32)
            n315 = global read "GlobalVI.vi" "emergencyStop"() -> (w1021:bool)
            n316 = Greater?(x=w1014, y=u32 10000) -> (0:w1015:bool)
            n317 = local read "liftState"() -> (w1019:i32)
            n318 = local write "timeoutCounter"(w1014) -> ()
            n319 = local write "timeoutError"(w1015) -> ()
            n320 = Not Equal?(x=w1019, y=3 ("liftState")) -> (x != y?=w1020:bool)
            n321 = Or(x=w1021, y=w1020) -> (x .or. y?=w1017:bool)
          }
          n322 = call "Time Delay 7"("error in (no error)"=w1004, "Delay Time (s)"=2.0) -> ("error out"=w1001:errorcluster)  [unwired: 9 in]
          n323 = case shown="True" w999 {
            tunnel: w1001 -> [_ _]
            tunnel: w1000 -> [w1008 _]
            frame False {
              n324 = case shown="True" w1008 {
                frame True {
                  w1009 = 0 ("PickingRoutine")
                  n325 = global write "GlobalVI.vi" "PickingRoutine"(w1009) -> ()
                  n326 = local write "liftState"(w1009) -> ()
                }
                frame False {
                  n327 = local read "liftState"() -> (w1010:i32)
                  n328 = Increment(x=w1010) -> (x+1=w1011:i32)
                  n329 = local write "liftState"(w1011) -> ()
                }
              }
            }
            frame True {
              n330 = global write "GlobalVI.vi" "PickingRoutine"(3 ("PickingRoutine")) -> ()
              n331 = local write "liftState"(0 ("liftState")) -> ()
            }
          }
        }
        frame 4 {
          n332 = global write "GlobalVI.vi" "currentLiftState"(w1124) -> ()
          n333 = while {
            tunnel: [w1206] -> w1125
            tunnel: [w1197] -> w1122
            tunnel: [w1194] -> w1123
            stop <- w1207 stop-if-true
            n334 = global read "GlobalVI.vi" "emergencyStop"() -> (w1199:bool)
            n335 = global read "GlobalVI.vi" "PickingRoutine"() -> (w1195:i32)
            n336 = xnode "Sensor 10"() -> ("B/DIO10 (Pin 31)"=w1202:bool)  [unwired: 1 in, 1 out]
            "B/DIO10 (Pin 31) - Sensor 5\nBackwards 3" <- w1202
            n337 = Equal?(x=w1195, y=0) -> (x = y?=w1200:bool)
            n338 = call "Motor_Controller.vi"("motorSelect"=enum16{"Motor A", "Motor B"}."Motor B", "direction"=enum16{"Forward", "Backward"}."Backward", "stopMotors"=FALSE) -> ("error out"=w1206:errorcluster)  [unwired: 12 in]
            n339 = Equal?(x=w1195, y=3) -> (x = y?=w1194:bool)
            n340 = Or(x=w1199, y=w1200) -> (x .or. y?=w1197:bool)
            n341 = Or(x=w1197, y=w1194) -> (x .or. y?=w1196:bool)
            n342 = Or(x=w1202, y=w1196) -> (x .or. y?=w1207:bool)
          }
          n343 = while {
            tunnel: TRUE ("COMM (Red)") -> [w1157]
            stop <- w1147 stop-if-true
            n344 = global read "GlobalVI.vi" "emergencyStop"() -> (w1148:bool)
            n345 = feedback #8(FALSE) -> (w1155:bool)
            n346 = Exclusive Or(1:w1157, 2:w1155) -> (0:w1156:bool)
            n347 = feedback-in #8(w1156) -> ()
            n348 = local read "liftState"() -> (w1150:i32)
            n349 = xnode "Running LED 8"("CommG"=w1155, "CommR"=TRUE) -> ("error out"=w1152:errorcluster)  [unwired: 1 in]
            n350 = Not Equal?(x=w1150, y=4 ("liftState")) -> (x != y?=w1149:bool)
            n351 = Or(x=w1148, y=w1149) -> (x .or. y?=w1147:bool)
            n352 = call "Time Delay8"("error in (no error)"=w1152, "Delay Time (s)"=0.25) -> ()  [unwired: 9 in, 1 out]
          }
          n353 = call "Motor_Controller.vi"("error in (no error)"=w1125, "stopMotors"=TRUE) -> ("error out"=w1126:errorcluster)  [unwired: 13 in]
          n354 = while {
            stop <- w1139 stop-if-true
            n355 = Tick Count (ms)() -> (millisecond timer value=w1145:u32)
            n356 = local read "timerCount"() -> (w1144:u32)
            n357 = global read "GlobalVI.vi" "emergencyStop"() -> (w1143:bool)
            n358 = Subtract(x=w1145, y=w1144) -> (x-y=w1136:u32)
            n359 = local read "liftState"() -> (w1141:i32)
            n360 = Greater?(x=w1136, y=u32 10000) -> (0:w1137:bool)
            n361 = Not Equal?(x=w1141, y=4 ("liftState")) -> (x != y?=w1142:bool)
            n362 = local write "timeoutCounter"(w1136) -> ()
            n363 = local write "timeoutError"(w1137) -> ()
            n364 = Or(x=w1143, y=w1142) -> (x .or. y?=w1139:bool)
          }
          n365 = call "Time Delay 8"("error in (no error)"=w1126, "Delay Time (s)"=1.0) -> ("error out"=w1121:errorcluster)  [unwired: 9 in]
          n366 = case shown="False" w1123 {
            tunnel: w1122 -> [w1130 _]
            tunnel: w1121 -> [_ _]
            frame False {
              n367 = case shown="False" w1130 {
                frame False {
                  n368 = local read "liftState"() -> (w1132:i32)
                  n369 = Increment(x=w1132) -> (x+1=w1131:i32)
                  n370 = local write "liftState"(w1131) -> ()
                }
                frame True {
                  w1133 = 0 ("PickingRoutine")
                  n371 = global write "GlobalVI.vi" "PickingRoutine"(w1133) -> ()
                  n372 = local write "liftState"(w1133) -> ()
                }
              }
            }
            frame True {
              n373 = global write "GlobalVI.vi" "PickingRoutine"(3 ("PickingRoutine")) -> ()
              n374 = local write "liftState"(0 ("liftState")) -> ()
            }
          }
        }
      }
    }
    event "CancelBin": Value Change {
      # "Cancel state"
      n375 = event-data() -> ()  [unwired: 1 in, 6 out]
      n376 = global read "GlobalVI.vi" "CancelBin"() -> (→"CancelBin":bool)
      n377 = flat-sequence {
        tunnel: [w1247] -> w1244
        tunnel: [w1296] -> w1243
        tunnel: w1244 -> [w1295]
        tunnel: w1243 -> [w1393]
        frame #0 {
          # "Stop and disable motors"
          n378 = xnode "Disable Motors 4"("IN1 (B/DIO1 (Pin 13))"=FALSE ("IN2 (B/DIO1 (Pin 13))"), "IN2 (B/DIO2 (Pin 15))"=FALSE ("IN3 (B/DIO2 (Pin 15))"), "IN3 (B/DIO4 (Pin 19))"=FALSE ("IN4 (B/DIO3 (Pin 17))"), "IN4 (B/DIO3 (Pin 17))"=FALSE ("ENABLE A (B/DIO13 (Pin 26))"), "ENABLE A (B/DIO0 (Pin 11))"=FALSE ("ENABLE B (B/DIO8 (Pin 27))"), "ENABLE B (B/DIO5 (Pin 21))"=FALSE ("ENABLE B (B/DIO8 (Pin 27))")) -> ("error out"=w1248:errorcluster)  [unwired: 1 in]
          n379 = call "Time Delay9"("error in (no error)"=w1248, "Delay Time (s)"=0.5) -> ("error out"=w1247:errorcluster)  [unwired: 9 in]
        }
        frame #1 {
          # "Move lift to home position."
          n380 = while {
            tunnel: [w1350] -> w1304
            tunnel: w1295 -> [w1349]
            stop <- w1351 stop-if-true
            n381 = global read "GlobalVI.vi" "emergencyStop"() -> (w1353:bool)
            n382 = xnode "Sensor 6"() -> ("B/DIO7 (Pin 25)"=w1352:bool)  [unwired: 1 in, 1 out]
            "B/DIO7 (Pin 25) 2" <- w1352
            n383 = call "Motor_Controller.vi"("error in (no error)"=w1349, "motorSelect"=enum16{"Motor A", "Motor B"}."Motor A", "direction"=enum16{"Forward", "Backward"}."Backward", "stopMotors"=FALSE) -> ("error out"=w1350:errorcluster)  [unwired: 11 in]
            n384 = Or(x=w1352, y=w1353) -> (x .or. y?=w1351:bool)
          }
          n385 = call "Motor_Controller.vi"("error in (no error)"=w1304, "stopMotors"=TRUE) -> ("error out"=w1302:errorcluster)  [unwired: 13 in]
          n386 = call "Time Delay10"("error in (no error)"=w1302, "Delay Time (s)"=1.0) -> ("error out"=w1301:errorcluster)  [unwired: 9 in]
          n387 = while {
            tunnel: w1301 -> [w1310]
            tunnel: [w1306] -> w1300
            stop <- w1307 stop-if-true
            n388 = xnode "Sensor"() -> ("B/DIO10 (Pin 31)"=w1308:bool)  [unwired: 1 in, 1 out]
            "B/DIO10 (Pin 31) 2" <- w1308
            n389 = global read "GlobalVI.vi" "emergencyStop"() -> (w1309:bool)
            n390 = call "Motor_Controller.vi"("error in (no error)"=w1310, "motorSelect"=enum16{"Motor A", "Motor B"}."Motor B", "direction"=enum16{"Forward", "Backward"}."Backward", "stopMotors"=FALSE) -> ("error out"=w1306:errorcluster)  [unwired: 11 in]
            n391 = Or(x=w1308, y=w1309) -> (x .or. y?=w1307:bool)
          }
          n392 = call "Motor_Controller.vi"("error in (no error)"=w1300, "stopMotors"=TRUE) -> ("error out"=w1298:errorcluster)  [unwired: 13 in]
          n393 = call "Time Delay11"("error in (no error)"=w1298, "Delay Time (s)"=0.5) -> ("error out"=w1296:errorcluster)  [unwired: 9 in]
        }
        frame #2 {
          w1392 = 0 ("PickingRoutine")
          # "Set lift to default state\nand wait for another \ncommand from TX2"
          n394 = global write "GlobalVI.vi" "PickingRoutine"(w1392) -> ()
          n395 = xnode "Disable Motors 5"("IN1 (B/DIO1 (Pin 13))"=FALSE ("IN2 (B/DIO1 (Pin 13))"), "IN2 (B/DIO2 (Pin 15))"=FALSE ("IN3 (B/DIO2 (Pin 15))"), "IN3 (B/DIO4 (Pin 19))"=FALSE ("IN4 (B/DIO3 (Pin 17))"), "IN4 (B/DIO3 (Pin 17))"=FALSE ("ENABLE A (B/DIO13 (Pin 26))"), "ENABLE A (B/DIO0 (Pin 11))"=FALSE ("ENABLE B (B/DIO8 (Pin 27))"), "ENABLE B (B/DIO5 (Pin 21))"=FALSE ("ENABLE B (B/DIO8 (Pin 27))"), "error in (no error)"=w1393) -> ()  [unwired: 1 out]
          n396 = local write "liftState"(w1392) -> ()
        }
      }
    }
  }
